vi "Init.vi"(8 "error in (no error)":errorcluster, 10 "ID":string, 11 "Deck in":refnum<class "Sample.lvclass">) -> (0 "error out":errorcluster, 3 "Deck out":refnum<class "Sample.lvclass">)   [LabVIEW 2020, in "Sample.lvclass"]
uses:
  Sample.lvclass
  Libraries/Track Info/Track Info.ctl
  State.ctl
  Sample.lvclass/Sample.ctl
  Packed Libraries/Globals.lvlibp/Constants.vi
  Packed Libraries/Messaging.lvlibp
  Packed Libraries/Globals.lvlibp
  Libraries/Track Info/Track Info.lvlib
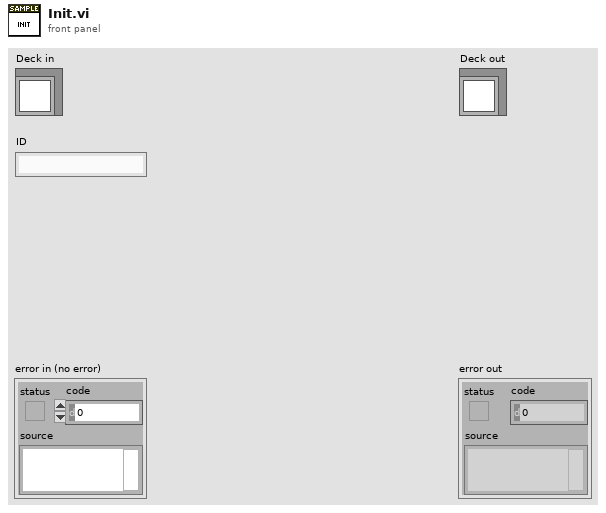
[diagram p1: front panel]
types:
  T1 = typedef "Track Info.lvlib/Track Info.ctl" = cluster{"Path":path, "Length (Samples)":i32, "Channels":i32, "Sample Rate (Hz)":i32, "BPM":dbl, "Cue Points (Samples)":i32[]}
  T2 = typedef "Sample.lvclass/State.ctl" = enum16{"No Track", "Loading", "Active", "Scratching", "Brake", "Backspin"}
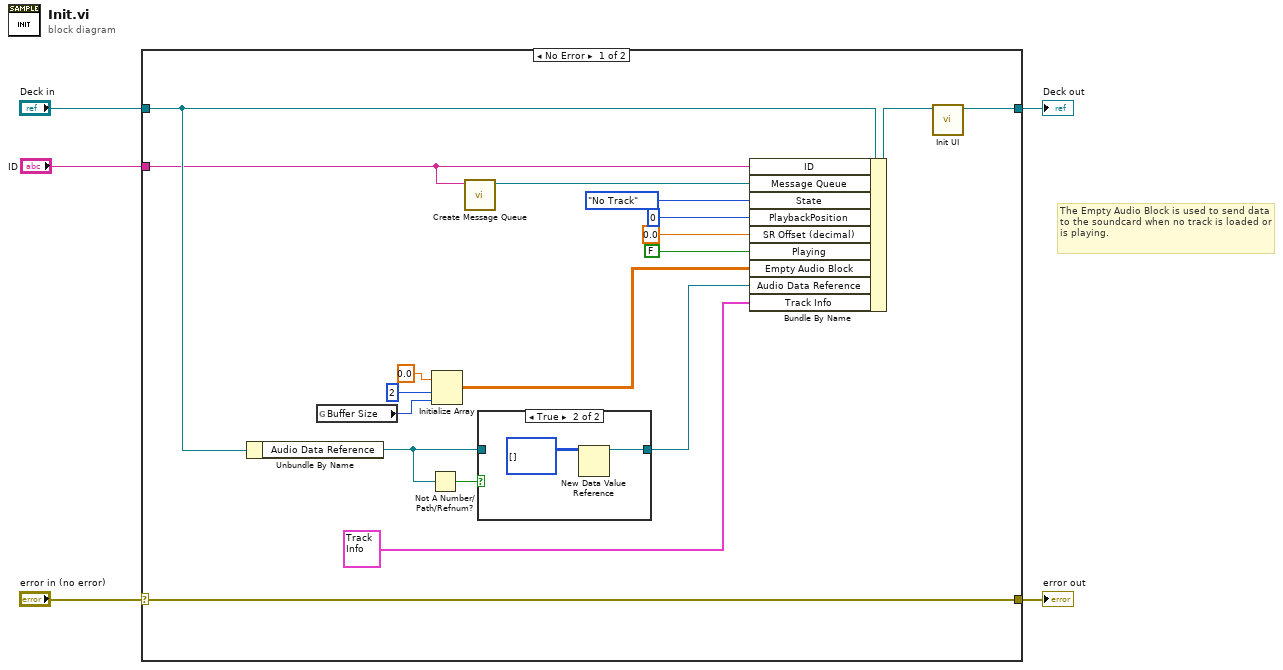
[diagram p0: block diagram]
diagram:
  # "The Empty Audio Block is used to send data to the soundcard when no track is loaded or is playing."
  n1 = case shown="No Error" "error in (no error)" {
    selector: "error in (no error)" -> [w23 w28]
    tunnel: [w23 w28] -> w4
    tunnel: [w7 w27] -> w2
    tunnel: "Deck in" -> [w18 w27]
    tunnel: "ID" -> [w12 _]
    frame No Error {
      n2 = Unbundle By Name(w18) -> ("Audio Data Reference"=w15:refnum<data-value>)
      n3 = global read "Constants.vi" "Buffer Size"() -> (w10:i32)
      n4 = Not A Number/Path/Refnum?(number/path/refnum=w15) -> (NaN/Path/Refnum?=w17:bool)
      n5 = Initialize Array(0.0, 2 ("dimension size"), w10) -> (w19:dbl[][])
      n6 = call "Create Message Queue.vi"("Queue Name"=w12) -> ("queue out"=w11:refnum<queue>)  [unwired: 9 in, 1 out]
      n7 = case shown="True" w17 {
        tunnel: [w24 w26] -> w16
        tunnel: w15 -> [w24 _]
        frame False {
        }
        frame True {
          n8 = New Data Value Reference(data value=i16[][] [] ("Audio Data")) -> (data value reference=w26:refnum<data-value>)  [unwired: 1 in, 1 out]
        }
      }
      n9 = Bundle By Name(cluster=w18, "ID"=w12, "Message Queue"=w11, "State"=State."No Track", "PlaybackPosition"=0 ("Playback Position (Samples)"), "SR Offset (decimal)"=0.0, "Playing"=FALSE ("PitchBendDown"), "Empty Audio Block"=w19, "Audio Data Reference"=w16, "Track Info"=T1 {"Path"=path "", "Length (Samples)"=0, "Channels"=0, "Sample Rate (Hz)"=0, "BPM"=0.0, "Cue Points (Samples)"=[-2147483648, -2147483648, -2147483648]}) -> (w8:refnum<class "Sample.lvclass">)
      n10 = call "Init UI.vi"("Deck in"=w8) -> ("Deck out"=w7:refnum<class "Sample.lvclass">)  [unwired: 9 in, 1 out]
    }
    frame Error {
    }
  }
  "error out" <- w4
  "Deck out" <- w2
